vi "Write Json.vi"(8 "Error In":errorcluster, 10 "JSON File Content":string, 11 "JSON File Name":string) -> (0 "Error Out":errorcluster)   [LabVIEW 2019, in "Asset.lvclass"]
uses:
  Asset.lvclass
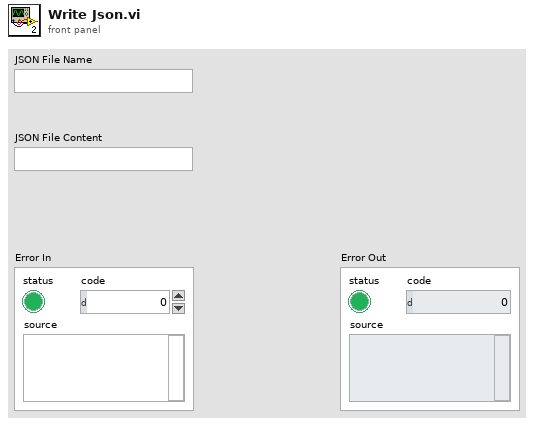
[diagram p1: front panel]
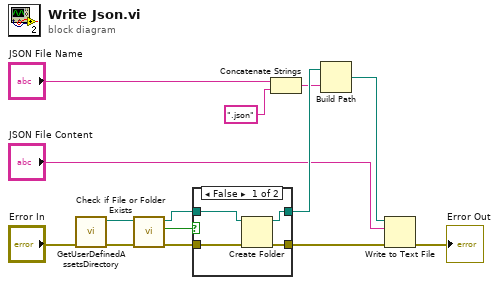
[diagram p0: block diagram]
diagram:
  n1 = call "GetUserDefinedAssetsDirectory.vi"("Error In"="Error In") -> ("Error Out"=w2:errorcluster, "User Defined Assets Directory"=w3:path)  [unwired: 9 in]
  n2 = call <vilib>:"Check if File or Folder Exists.vi"("error in (no error)"=w2, "path"=w3) -> ("error out"=w11:errorcluster, "file or folder exists?"=w14:bool, "dup path"=w13:path)  [unwired: 7 in]
  n3 = case shown="False" w14 {
    tunnel: w13 -> [w18 w20]
    tunnel: [w17 w20] -> w12
    tunnel: w11 -> [w16 w19]
    tunnel: [w15 w19] -> w10
    frame False {
      n4 = Create Folder(path (use dialog)=w18, error in=w16) -> (created path=w17:path, error out=w15:errorcluster)  [unwired: 1 in, 1 out]
    }
    frame True {
    }
  }
  n5 = Concatenate Strings("JSON File Name", ".json" ("string")) -> (w4:string)
  n6 = Build Path(base path=w12, name or relative path=w4) -> (appended path=w8:path)
  n7 = Write to Text File(file (use dialog)=w8, text="JSON File Content", error in=w10) -> (error out=→"Error Out":errorcluster)  [unwired: 1 in, 2 out]
